vi "Ascan.vi"(8 "error in (no error)":cluster{"状态":bool, "代码":i32, "源":string} caption="错误输入（无错误）") -> (0 "error out":cluster{"状态":bool, "代码":i32, "源":string} caption="错误输出")   [LabVIEW 2015, in "Debug.lvlib"]
uses:
  Debug.lvlib
  Support/Debug Ascan UI Data.ctl
  Support/Ascan Configuration.ctl
  Sub VIs/DAQ/DAQ Configuration.ctl
  Sub VIs/Digital Signal Processing/Support/DSP Configuration.ctl
  <vilib>/Analysis/3filter.llb/Filter Passband Type.ctl
  <vilib>/Analysis/4window.llb/windowTd.ctl
  Sub VIs/Boimetry Processing/Controls/Biometry Configuration.ctl
  support/Message Queue/Enqueue Message (Single).vi
  <vilib>/Utility/error.llb/Error Cluster From Error Code.vi
  <vilib>/ErrorRing/Error Ring.xnode
  support/Message Queue/Message Queue.lvlib
  support/User Event - Stop/User Event - Stop.lvlib
  Sub VIs/DAQ/DAQ.lvlib
  <vilib>/Analysis/NI_AALBase.lvlib
  <vilib>/Analysis/NI_AALPro.lvlib
  Sub VIs/Digital Signal Processing/Digital Signal Processing.lvlib
  Sub VIs/Boimetry Processing/Boimetry Processing.lvlib
  Settings/Settings.lvlib
panel:
  in  "退出":bool
  in  "停止按钮":bool
  in  "计算距离":bool
  in  "保存按钮":bool
  in  "开始":bool
  in  "nd":dbl
  out "Thickness":dbl
  out "Position":dbl
  out "processing":dbl[](graph)
  out "original":i16[](graph)
  out "状态栏":string
  in  "Settings":bool
  in  "Liquid Len":bool
  in  "DSP Change":enum16{"1st", "2nd"}(ring)
  in  "WLED":bool
  in  "IRLED2":bool
  in  "IRLED1":bool
  in  "Motor":bool
  in  "SLD":bool
  # "Ascan Setting"
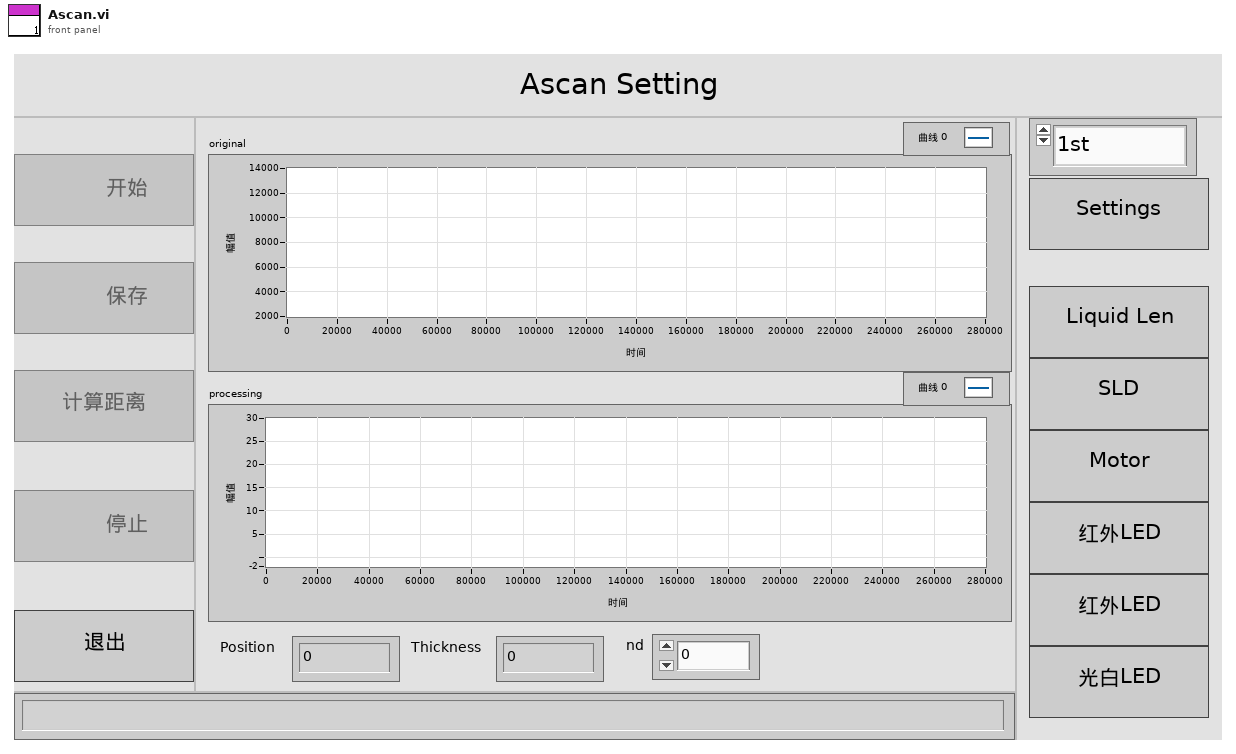
[diagram p1: front panel]
types:
  T1 = typedef "Debug.lvlib/Ascan Configuration.ctl" = cluster{"DAQ Configuration":T2, "DSP Parameter":T3, "Biometry Configuration":T6}
  T2 = typedef "DAQ.lvlib/DAQ Configuration.ctl" = cluster{"hDevice":i32, "DevNum":u8, "Configuration Parameter":i32[], "READ_MAX_LEN":i32, "DO":bool[]}
  T3 = typedef "Digital Signal Processing.lvlib/DSP Configuration.ctl" = cluster{"Sampling Frequency":dbl, "filter type":T4, "RF Filter Low Frequency":dbl, "RF Filter High Frequency":dbl, "RF Filter Taps":i32, "window":T5, "RF window parameter":dbl, "filter type 2":T4, "Demodulated Filter Low Frequency":dbl, "Demodulated Filter HighFrequency":dbl, "Demodulated Filter Order":i32, "SPAN":i32, "Logarithmic Base":dbl, "Noise path":string, "Work position parameter":i32[]}
  T4 = typedef "NI_AALBase.lvlib/Filter Passband Type.ctl" = enum32{"Lowpass", "Highpass", "Bandpass", "Bandstop"}
  T5 = typedef "NI_AALPro.lvlib/windowTd.ctl" = u32
  T6 = typedef "Boimetry Processing.lvlib/Biometry Configuration.ctl" = cluster{"Interference Width":i32, "Interference Threshold":dbl, "Cornea Len Division":i32, "Correction Data 1st Path":string, "1st_Start_Position":dbl, "Correction Data 2nd Path":string, "2nd_Start_Position":dbl, "Index Corneal":dbl, "Index Water":dbl, "Index Len":dbl, "Working Position":cluster{"FirstStart":i32, "FirstEnd":i32, "SecondStart":i32, "SecondEnd":i32}}
  T7 = typedef "Debug.lvlib/Debug Ascan UI Data.ctl" = cluster{"开始按钮引用句柄":refnum<vi>, "保持按钮引用句柄":refnum<vi>, "计算距离按钮l引用句柄":refnum<vi>, "停止按钮引用句柄":refnum<vi>, "状态栏引用句柄":refnum<vi>, "消息栏引用句柄":refnum<vi>, "退出按钮引用句柄":refnum<vi>, "SLD":refnum<vi>, "Motor":refnum<vi>}
  T8 = typedef "Message Queue.lvlib/All Message Queues Ascan.ctl" = cluster{"UI":refnum<queue>, "DAQ":refnum<queue>, "DSP":refnum<queue>, "CDL":refnum<queue>}
  T9 = typedef "Settings.lvlib/Settings.ctl" = cluster{"DAQ Configuration":T2, "DSP Configuration":T3, "Biometry Configuration":T6}
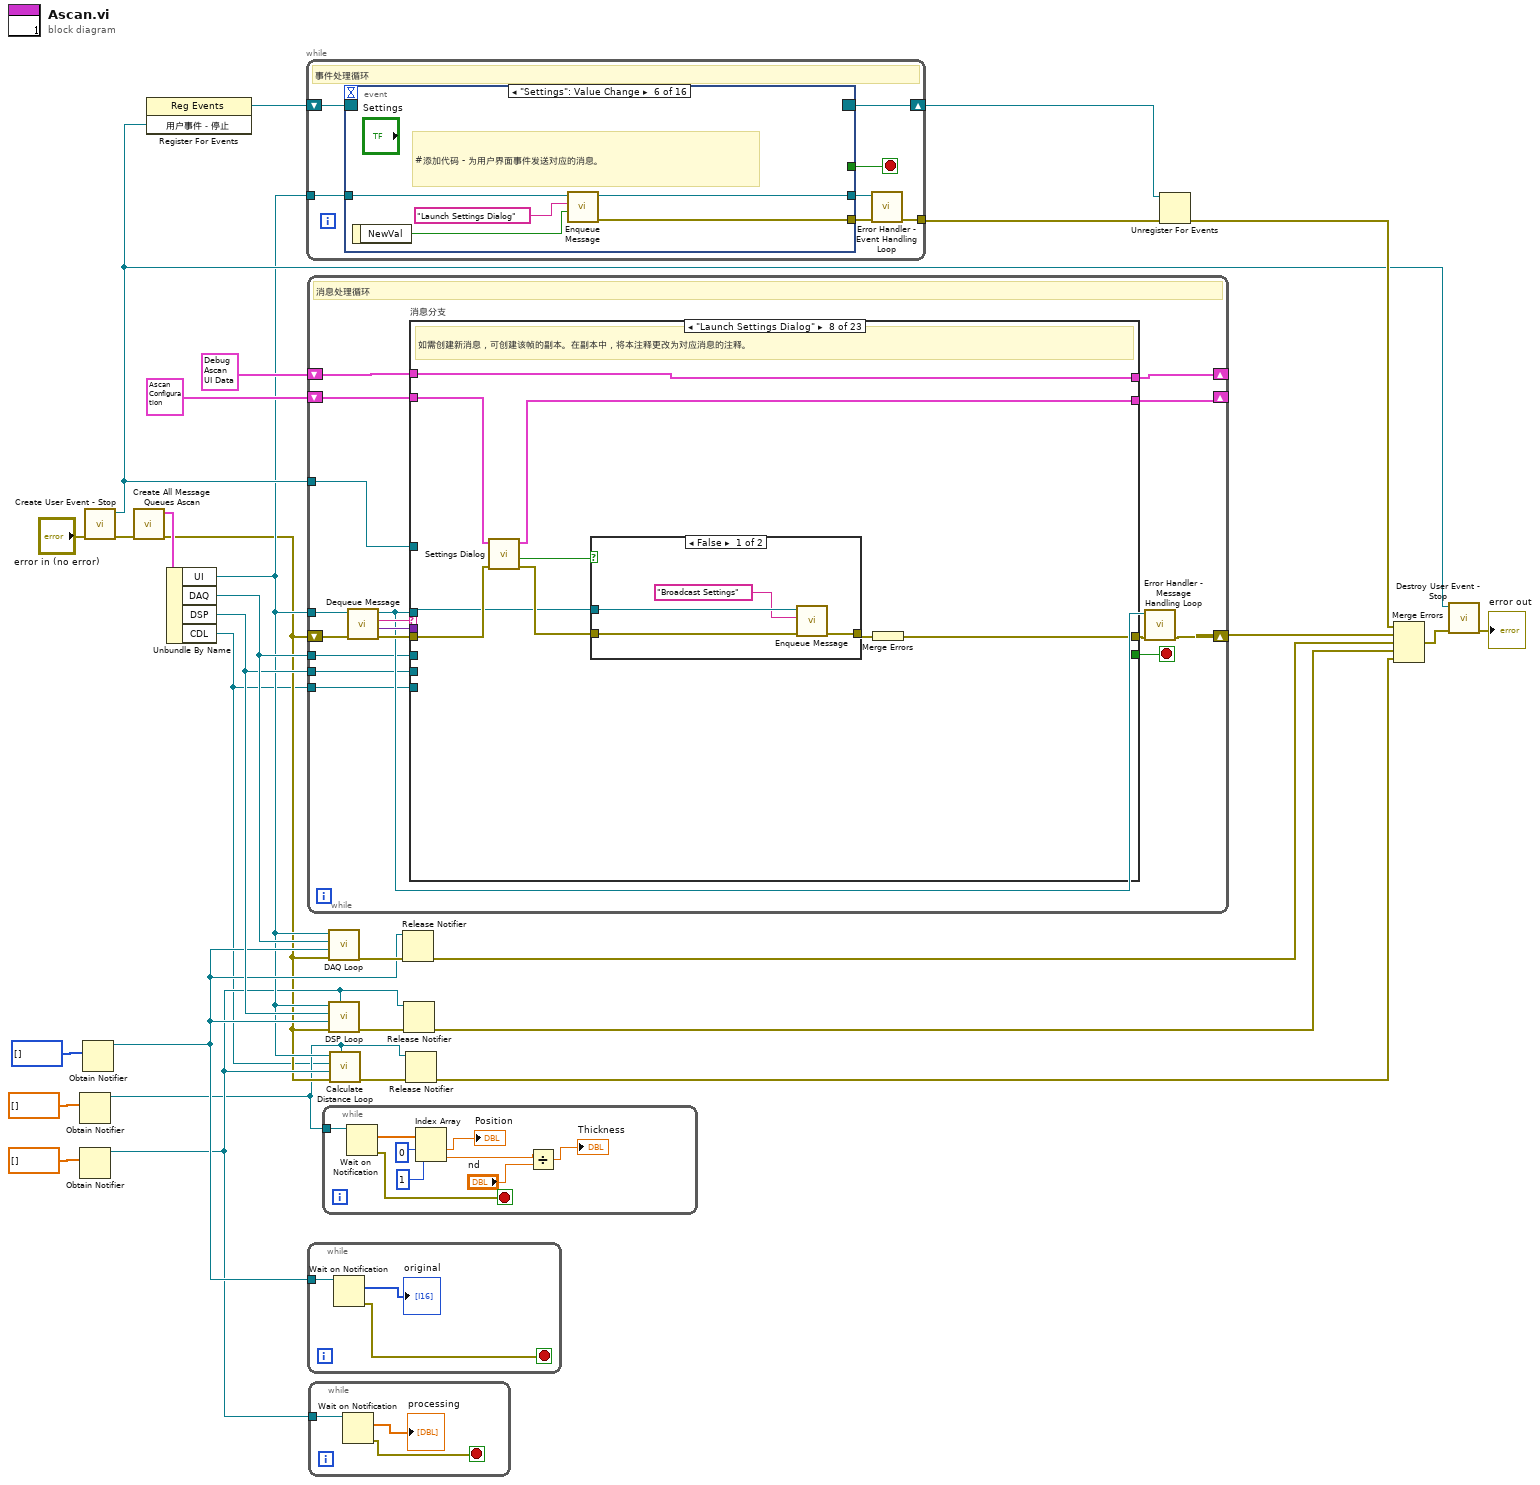
[diagram p0: block diagram]
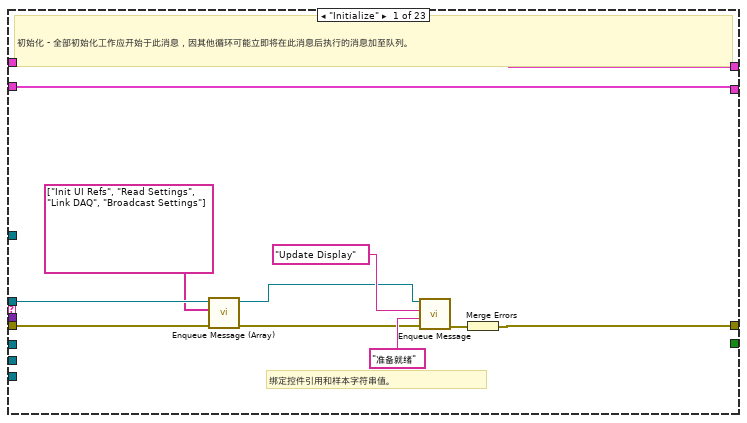
[diagram p2: hidden frame]
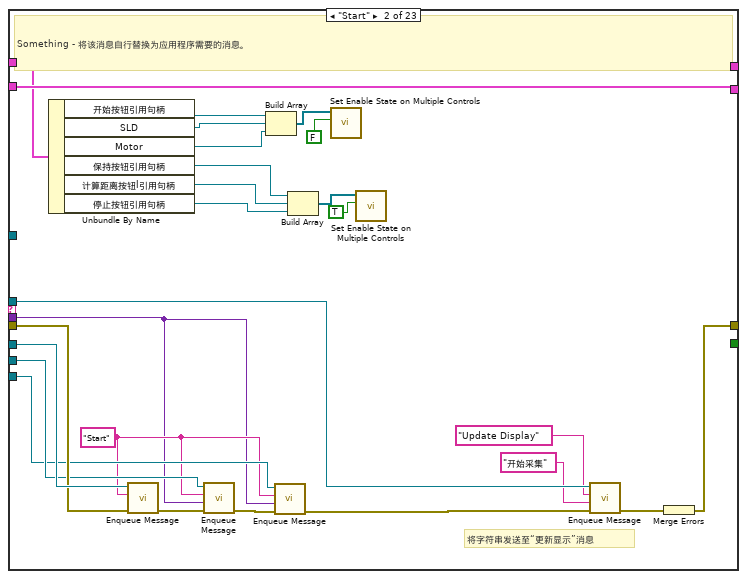
[diagram p3: hidden frame]
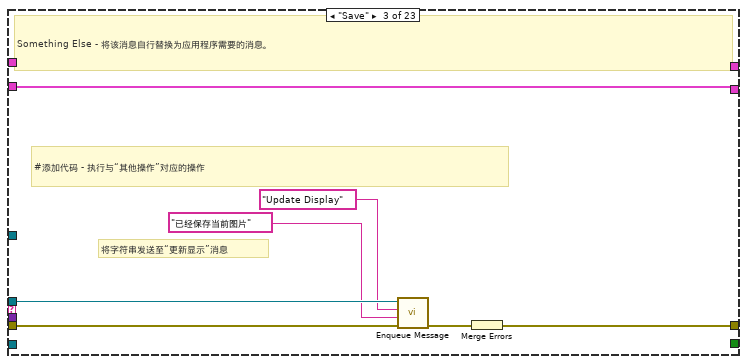
[diagram p4: hidden frame]
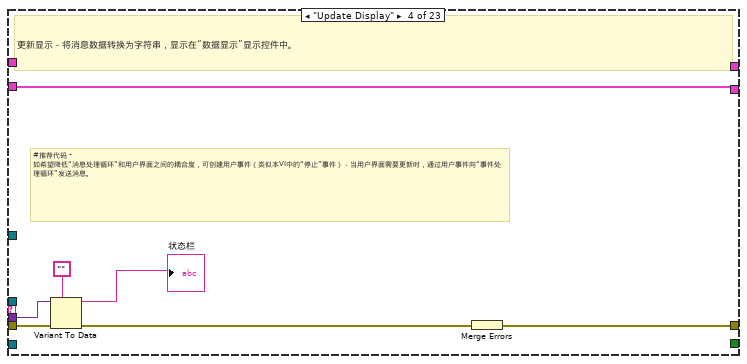
[diagram p5: hidden frame]
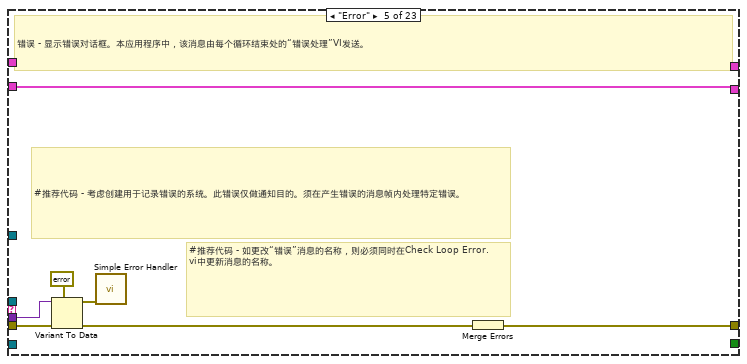
[diagram p6: hidden frame]
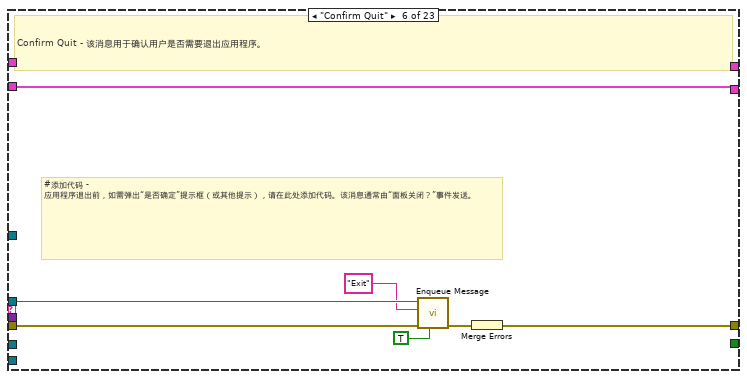
[diagram p7: hidden frame]
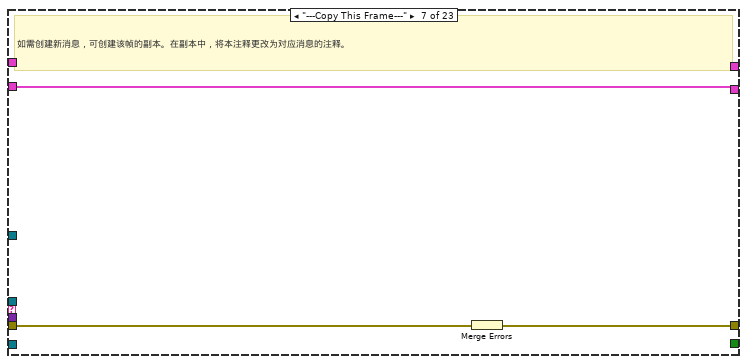
[diagram p8: hidden frame]
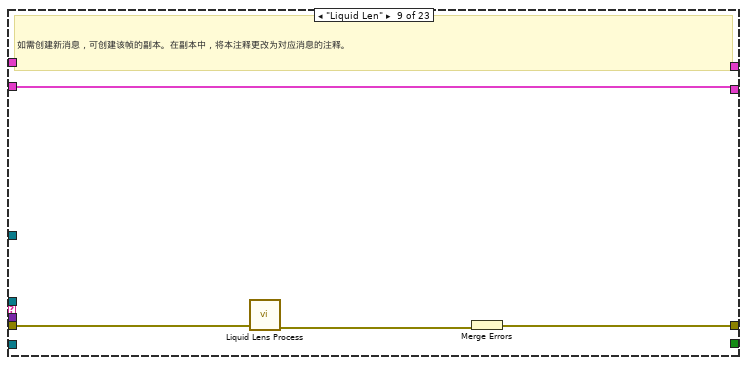
[diagram p10: hidden frame]
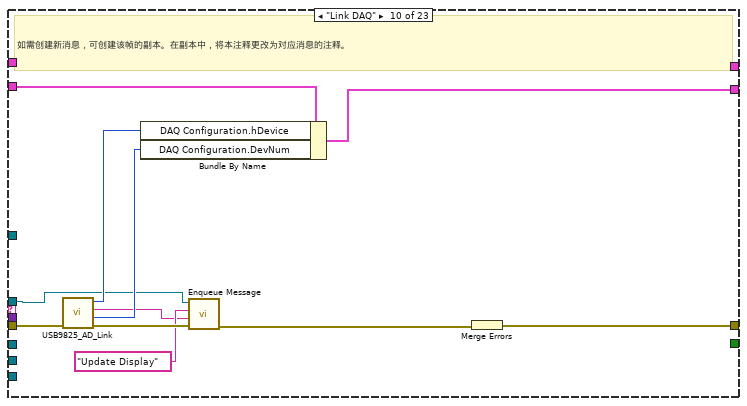
[diagram p11: hidden frame]
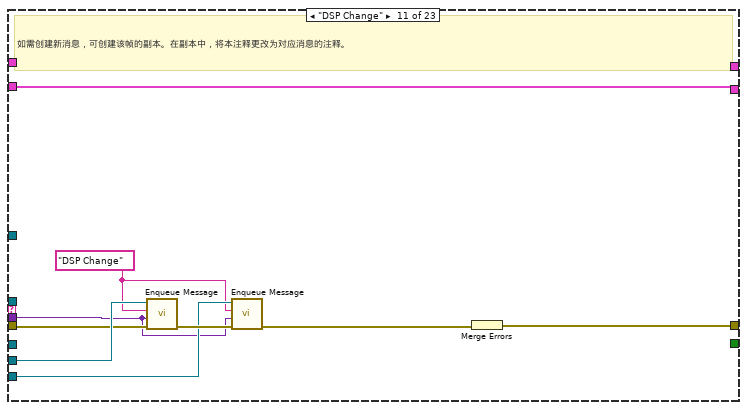
[diagram p12: hidden frame]
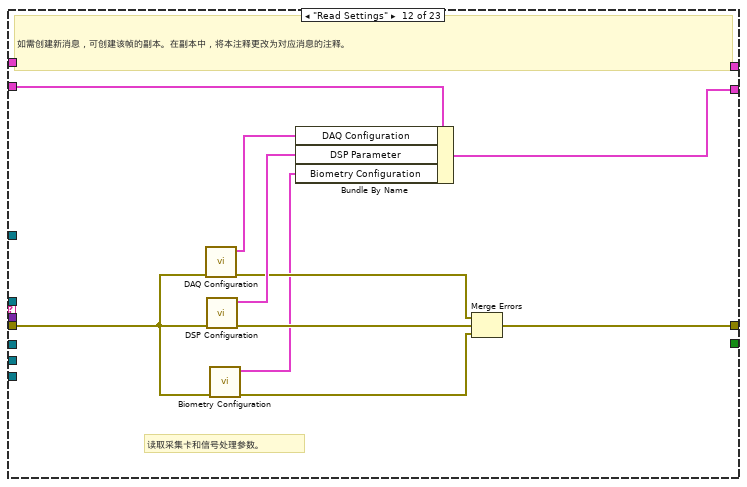
[diagram p13: hidden frame]
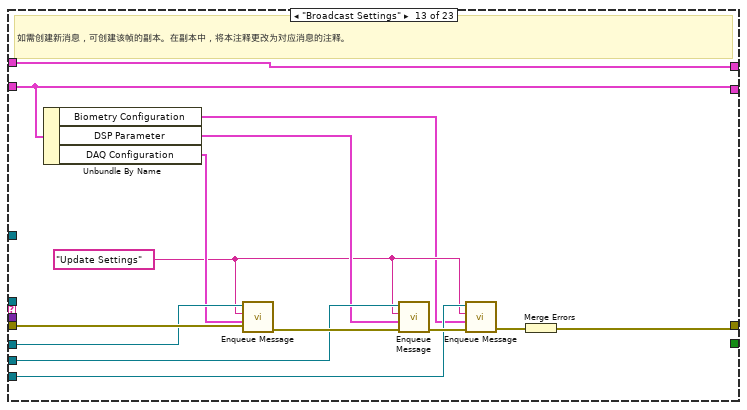
[diagram p14: hidden frame]
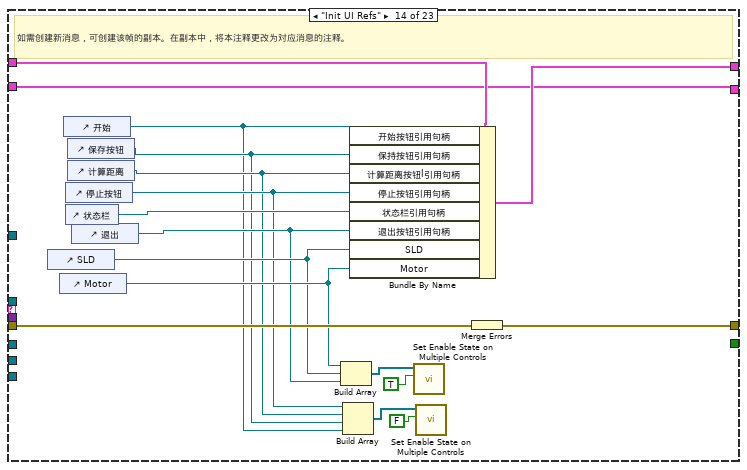
[diagram p15: hidden frame]
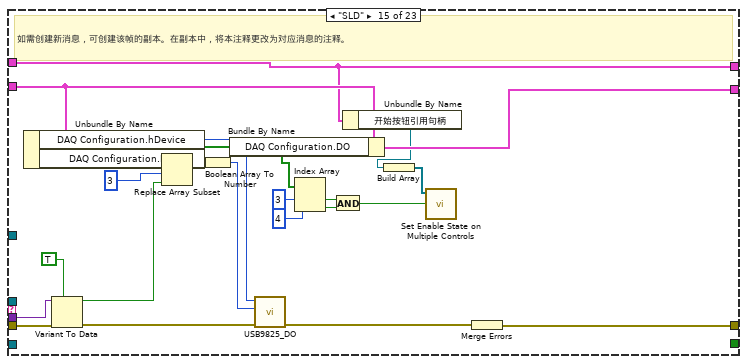
[diagram p16: hidden frame]
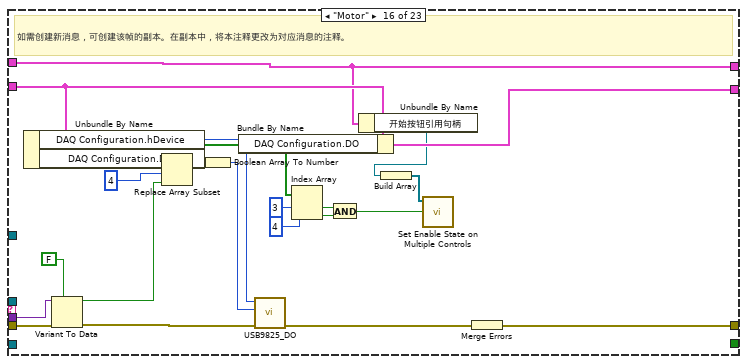
[diagram p17: hidden frame]
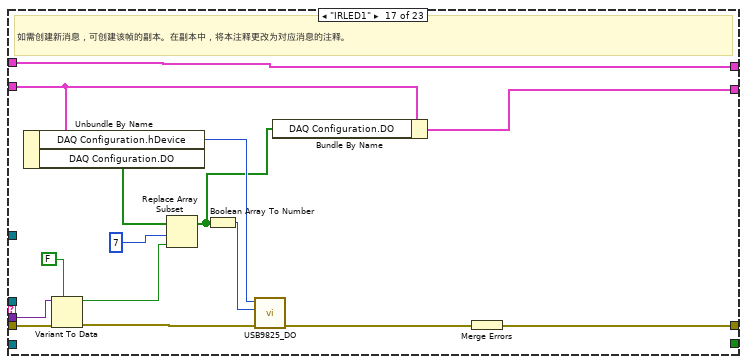
[diagram p18: hidden frame]
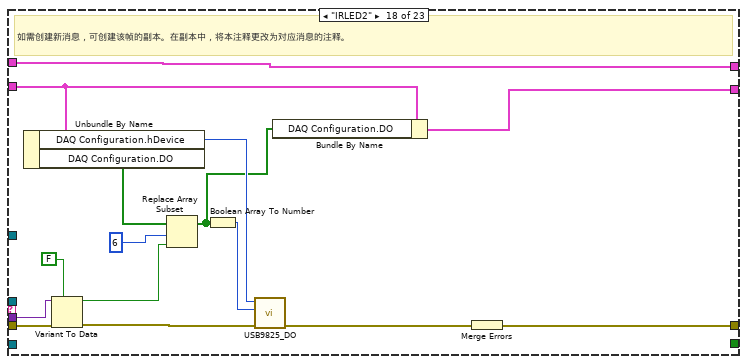
[diagram p19: hidden frame]
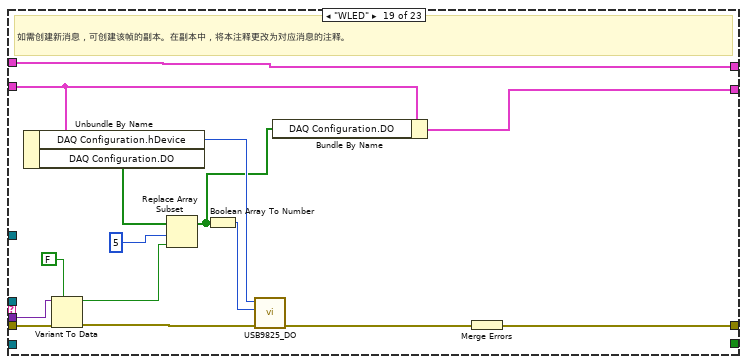
[diagram p20: hidden frame]
diagram:
  n1 = Obtain Notifier(notification data type=dbl[] []) -> (notifier out=w3:refnum<notifier>)  [unwired: 3 in, 2 out]
  n2 = Obtain Notifier(notification data type=dbl[] []) -> (notifier out=w7:refnum<notifier>)  [unwired: 3 in, 2 out]
  n3 = Obtain Notifier(notification data type=i16[] []) -> (notifier out=w12:refnum<notifier>)  [unwired: 3 in, 2 out]
  n4 = call "Create User Event - Stop.vi"("error in (no error)"="error in (no error)") -> ("error out"=w9:cluster{"状态":bool, "代码":i32, "源":string}, "用户事件－停止"=w25:refnum<user-event>)  [unwired: 9 in]
  n5 = call "Create All Message Queues Ascan.vi"("error in (no error)"=w9) -> ("error out"=w5:cluster{"状态":bool, "代码":i32, "源":string}, "消息队列"=w8:T8)  [unwired: 9 in]
  n6 = register-events(w25) -> (reference out=w30:refnum<event-registration>)  [unwired: 2 in, 1 out]
  n7 = Unbundle By Name(w8) -> ("UI"=w10:refnum<queue>, "DAQ"=w19:refnum<queue>, "DSP"=w14:refnum<queue>, "CDL"=w1:refnum<queue>)
  n8 = while {
    tunnel: w10 -> [w37]
    shift-right: [w35] -> w28
    shift-left: w30 -> [w36]
    tunnel: [w31] -> w29
    stop <- w33 stop-if-true
    # "事件处理循环"
    n9 = event shown="[5] \"Settings\": Value Change" {
      selector: w36 -> [_ _ _ _ _ _ _ _ _ _ _ _ _ _ _ _]
      dyn-events: [_ _ _ _ _ _ _ _ _ _ _ _ _ _ _ _] -> w35
      timeout: _ -> [_ _ _ _ _ _ _ _ _ _ _ _ _ _ _ _]
      tunnel: [_ _ _ _ _ _ _ _ _ _ _ _ _ _ _ TRUE ("Discard?")] -> w33
      tunnel: w37 -> [w43 w50 w56 w60 w65 w70 w75 w80 w85 w90 w95 w100 w102 w107 w112 w114]
      tunnel: [w40 _ w53 w57 w62 w67 w72 w77 w82 w87 w92 w99 _ w106 w111 _] -> w34
      tunnel: [w42 w49 w55 w59 w64 w69 w74 w79 w84 w89 w94 w98 w102 w105 w110 w114] -> w32
      event "开始": Value Change {
        n10 = event-data() -> ()  [unwired: 1 in, 1 out]
        n11 = local read "DSP Change"() -> (w39:enum16{"1st", "2nd"})
        n12 = case shown="\"2nd\"" w39 {
          tunnel: ["DSP 1st" ("Message") "DSP 2nd" ("Message")] -> w38
          frame "1st", Default {
          }
          frame "2nd" {
          }
        }
        n13 = call-poly "Enqueue Message.vi"("消息数据"=w38, "消息"="Start" ("Message"), "消息队列"=w43) -> ("error out"=w40:cluster{"状态":bool, "代码":i32, "源":string}, "消息队列副本"=w42:refnum<queue>)  [unwired: 7 in]
      }
      event "DSP Change": Value Change {
        n14 = event-data() -> ()  [unwired: 1 in, 1 out]
        n15 = case shown="\"2nd\"" "DSP Change" {
          tunnel: ["DSP 1st" ("Message") "DSP 2nd" ("Message")] -> w47
          frame "1st", Default {
          }
          frame "2nd" {
          }
        }
        n16 = call-poly "Enqueue Message.vi"("消息数据"=w47, "消息"="DSP Change", "消息队列"=w50) -> ("消息队列副本"=w49:refnum<queue>)  [unwired: 7 in, 1 out]
      }
      event "保存按钮": Value Change {
        # "#添加代码 - 为用户界面事件发送对应的消息。"
        n17 = event-data() -> ()  [unwired: 1 in, 1 out]
        n18 = call-poly "Enqueue Message.vi"("消息"="Save" ("Message"), "消息队列"=w56) -> ("error out"=w53:cluster{"状态":bool, "代码":i32, "源":string}, "消息队列副本"=w55:refnum<queue>)  [unwired: 8 in]
      }
      event "计算距离": Value Change {
        # "#添加代码 - 为用户界面事件发送对应的消息。"
        n19 = event-data() -> ()  [unwired: 1 in, 1 out]
        n20 = call-poly "Enqueue Message.vi"("消息"="Calculate" ("Message"), "消息队列"=w60) -> ("error out"=w57:cluster{"状态":bool, "代码":i32, "源":string}, "消息队列副本"=w59:refnum<queue>)  [unwired: 8 in]
      }
      event "SLD": Value Change {
        # "#添加代码 - 为用户界面事件发送对应的消息。"
        n21 = event-data() -> ("NewVal"=w61:bool)  [unwired: 1 in]
        n22 = call-poly "Enqueue Message.vi"("消息数据"=w61, "消息"="SLD" ("Message"), "消息队列"=w65) -> ("error out"=w62:cluster{"状态":bool, "代码":i32, "源":string}, "消息队列副本"=w64:refnum<queue>)  [unwired: 7 in]
      }
      event "Settings": Value Change {
        # "#添加代码 - 为用户界面事件发送对应的消息。"
        n23 = event-data() -> ("NewVal"=w66:bool)  [unwired: 1 in]
        n24 = call-poly "Enqueue Message.vi"("消息数据"=w66, "消息"="Launch Settings Dialog" ("Message"), "消息队列"=w70) -> ("error out"=w67:cluster{"状态":bool, "代码":i32, "源":string}, "消息队列副本"=w69:refnum<queue>)  [unwired: 7 in]
      }
      event "Motor": Value Change {
        # "#添加代码 - 为用户界面事件发送对应的消息。"
        n25 = event-data() -> ("NewVal"=w71:bool)  [unwired: 1 in]
        n26 = call-poly "Enqueue Message.vi"("消息数据"=w71, "消息"="Motor" ("Message"), "消息队列"=w75) -> ("error out"=w72:cluster{"状态":bool, "代码":i32, "源":string}, "消息队列副本"=w74:refnum<queue>)  [unwired: 7 in]
      }
      event "Liquid Len": Value Change {
        # "#添加代码 - 为用户界面事件发送对应的消息。"
        n27 = event-data() -> ("NewVal"=w76:bool)  [unwired: 1 in]
        n28 = call-poly "Enqueue Message.vi"("消息数据"=w76, "消息"="Liquid Len" ("Message"), "消息队列"=w80) -> ("error out"=w77:cluster{"状态":bool, "代码":i32, "源":string}, "消息队列副本"=w79:refnum<queue>)  [unwired: 7 in]
      }
      event "IRLED1": Value Change {
        # "#添加代码 - 为用户界面事件发送对应的消息。"
        n29 = event-data() -> ("NewVal"=w81:bool)  [unwired: 1 in]
        n30 = call-poly "Enqueue Message.vi"("消息数据"=w81, "消息"="IRLED1" ("Message"), "消息队列"=w85) -> ("error out"=w82:cluster{"状态":bool, "代码":i32, "源":string}, "消息队列副本"=w84:refnum<queue>)  [unwired: 7 in]
      }
      event "IRLED2": Value Change {
        # "#添加代码 - 为用户界面事件发送对应的消息。"
        n31 = event-data() -> ("NewVal"=w86:bool)  [unwired: 1 in]
        n32 = call-poly "Enqueue Message.vi"("消息数据"=w86, "消息"="IRLED2" ("Message"), "消息队列"=w90) -> ("error out"=w87:cluster{"状态":bool, "代码":i32, "源":string}, "消息队列副本"=w89:refnum<queue>)  [unwired: 7 in]
      }
      event "WLED": Value Change {
        # "#添加代码 - 为用户界面事件发送对应的消息。"
        n33 = event-data() -> ("NewVal"=w91:bool)  [unwired: 1 in]
        n34 = call-poly "Enqueue Message.vi"("消息数据"=w91, "消息"="WLED" ("Message"), "消息队列"=w95) -> ("error out"=w92:cluster{"状态":bool, "代码":i32, "源":string}, "消息队列副本"=w94:refnum<queue>)  [unwired: 7 in]
      }
      event Panel Close? {
        # "如用户关闭VI面板，则发送“确认退出”消息。丢弃事件，因此“确认退出”消息有运行时机。"
        n35 = event-data() -> ()  [unwired: 1 in, 1 out]
        n36 = call-poly "Enqueue Message.vi"("优先消息？ (F)"=TRUE ("Priority Message? (F)"), "消息"="Confirm Quit" ("Message"), "消息队列"=w100) -> ("error out"=w99:cluster{"状态":bool, "代码":i32, "源":string}, "消息队列副本"=w98:refnum<queue>)  [unwired: 7 in]
        n37 = event-data ("Event Filter Node")("Discard?"=TRUE) -> ()  [unwired: 1 in, 1 out]
      }
      event Application Instance Close {
        # "#推荐代码 - 当项目关闭时，项目的所有VI将被中止并从内存中释放。本事件帧内的所有代码都确保能够执行完成，因此可在此处添加必须执行的清理代码。"
        n38 = event-data() -> ()  [unwired: 1 in, 1 out]
      }
      event "停止按钮": Value Change {
        n39 = event-data() -> ()  [unwired: 1 in, 1 out]
        n40 = call-poly "Enqueue Message.vi"("优先消息？ (F)"=TRUE ("Priority Message? (F)"), "消息"="Stop" ("Message"), "消息队列"=w107) -> ("error out"=w106:cluster{"状态":bool, "代码":i32, "源":string}, "消息队列副本"=w105:refnum<queue>)  [unwired: 7 in]
      }
      event "退出": Value Change {
        n41 = event-data() -> ()  [unwired: 1 in, 1 out]
        n42 = call-poly "Enqueue Message.vi"("优先消息？ (F)"=TRUE ("Priority Message? (F)"), "消息"="Exit" ("Message"), "消息队列"=w112) -> ("error out"=w111:cluster{"状态":bool, "代码":i32, "源":string}, "消息队列副本"=w110:refnum<queue>)  [unwired: 7 in]
      }
      event User Event {
        (unwired) "“退出”按钮按下" ("VI Stopped")
        # "消息处理循环对“退出”消息进行处理，触发该事件，从而使事件处理循环停止运行。"
        n43 = event-data() -> ()  [unwired: 1 in, 1 out]
      }
    }
    n44 = call "Error Handler - Event Handling Loop.vi"("error in (no error)"=w34, "消息队列"=w32) -> ("错误输入副本"=w31:cluster{"状态":bool, "代码":i32, "源":string})  [unwired: 8 in, 1 out]
  }
  n45 = while {
    tunnel: w10 -> [w123]
    shift-right: [w130] -> _
    shift-left: T7 {"开始按钮引用句柄"=refnum, "保持按钮引用句柄"=refnum, "计算距离按钮l引用句柄"=refnum, "停止按钮引用句柄"=refnum, "状态栏引用句柄"=refnum, "消息栏引用句柄"=refnum, "退出按钮引用句柄"=refnum, "SLD"=refnum, "Motor"=refnum} ("UI数据") -> [w131]
    tunnel: w25 -> [w128]
    tunnel: w19 -> [w120]
    shift-right: [w118] -> _
    shift-left: T1 {"DAQ Configuration"={"hDevice"=0, "DevNum"=0, "Configuration Parameter"=[], "READ_MAX_LEN"=0, "DO"=[]}, "DSP Parameter"={"Sampling Frequency"=0.0, "filter type"=enum."Lowpass", "RF Filter Low Frequency"=0.0, "RF Filter High Frequency"=0.0, "RF Filter Taps"=0, "window"=0, "RF window parameter"=nan, "filter type 2"=enum."Lowpass", "Demodulated Filter Low Frequency"=0.0, "Demodulated Filter HighFrequency"=0.0, "Demodulated Filter Order"=0, "SPAN"=0, "Logarithmic Base"=0.0, "Noise path"="", "Work position parameter"=[]}, "Biometry Configuration"={"Interference Width"=0, "Interference Threshold"=0.0, "Cornea Len Division"=0, "Correction Data 1st Path"="", "1st_Start_Position"=0.0, "Correction Data 2nd Path"="", "2nd_Start_Position"=0.0, "Index Corneal"=0.0, "Index Water"=0.0, "Index Len"=0.0, "Working Position"={"FirstStart"=0, "FirstEnd"=0, "SecondStart"=0, "SecondEnd"=0}}} ("Ascan Configuration") -> [w119]
    tunnel: w14 -> [w117]
    shift-right: [w116] -> w18
    shift-left: w5 -> [w127]
    tunnel: w1 -> [w115]
    stop <- w129 stop-if-true
    # "消息处理循环"
    n46 = call "Dequeue Message.vi"("error in (no error)"=w127, "消息队列"=w123) -> ("error out"=w126:cluster{"状态":bool, "代码":i32, "源":string}, "消息数据"=w124:variant, "消息"=w125:string, "消息队列副本"=w122:refnum<queue>)  [unwired: 6 in]
    n47 = case "消息分支" shown="\"Launch Settings Dialog\"" w125 {
      selector: w125 -> [_ _ _ _ _ _ _ _ _ _ _ _ _ _ _ _ _ _ _ _ _ _ w420]
      tunnel: w122 -> [w137 w166 w172 _ _ w196 _ w206 _ w227 _ _ _ _ _ _ _ _ _ _ _ w418 _]
      tunnel: w126 -> [w134 w162 w174 w182 w192 w200 w204 w211 w220 w233 w241 w248 w268 w287 w308 w330 w345 w360 w375 w396 w401 w410 _]
      tunnel: [w139 w168 w175 w183 w186 w198 w202 w212 w222 w234 w244 w255 w269 w286 w309 w331 w346 w361 w376 w397 w399 w414 w421] -> w121
      tunnel: w131 -> [w138 w158 w176 w184 w191 w199 w203 w213 w223 w235 w245 w256 w270 w285 w291 w311 w332 w347 w362 w383 w400 w417 w422]
      tunnel: [w138 w158 w176 w184 w191 w199 w203 w213 w223 w235 w245 w256 w270 w284 w291 w311 w332 w347 w362 w383 w400 w417 w422] -> w130
      tunnel: [_ _ _ _ _ _ _ _ _ _ _ _ _ _ _ _ _ _ _ _ _ TRUE _] -> w129
      tunnel: w124 -> [_ w143 _ w181 w190 _ _ _ _ _ w236 _ _ _ w307 w329 w344 w359 w374 _ _ _ _]
      tunnel: w128 -> [_ _ _ _ _ _ _ _ _ _ _ _ _ _ _ _ _ _ _ _ _ w413 _]
      tunnel: w120 -> [_ w163 _ _ _ _ _ _ _ _ _ _ w267 _ _ _ _ _ _ w395 _ w411 _]
      tunnel: [w133 w161 w169 w177 w185 w193 w201 w209 w221 w224 w243 w251 w264 w271 w297 w319 w334 w349 w364 w394 w398 w409 w419] -> w118
      tunnel: w119 -> [w133 w161 w169 w177 w185 w193 w201 w210 w221 w232 w243 w252 w264 w271 w298 w320 w335 w350 w365 w394 w398 w409 w419]
      tunnel: w117 -> [_ w159 _ _ _ _ _ _ _ _ w242 _ w265 _ _ _ _ _ _ w392 _ w407 _]
      tunnel: w115 -> [_ w145 _ _ _ _ _ _ _ _ w238 _ w259 _ _ _ _ _ _ w378 _ w404 _]
      frame "Initialize" {
        # "绑定控件引用和样本字符串值。"
        # "初始化 - 全部初始化工作应开始于此消息，因其他循环可能立即将在此消息后执行的消息加至队列。"
        n48 = call "Enqueue Message (Array).vi"("error in (no error)"=w134, "消息数组"=string[] ["Init UI Refs", "Read Settings", "Link DAQ", "Broadcast Settings"], "消息队列"=w137) -> ("error out"=w132:cluster{"状态":bool, "代码":i32, "源":string}, "消息队列副本"=w136:refnum<queue>)  [unwired: 7 in]
        n49 = call-poly "Enqueue Message.vi"("error in (no error)"=w132, "消息数据"="准备就绪" ("Initial Message"), "消息"="Update Display" ("Message"), "消息队列"=w136) -> ("error out"=w140:cluster{"状态":bool, "代码":i32, "源":string})  [unwired: 6 in, 1 out]
        n50 = Merge Errors(w140) -> (w139:errorcluster)
      }
      frame "Start" {
        w144 = "Start" ("消息")
        # "将字符串发送至“更新显示”消息"
        # "Something - 将该消息自行替换为应用程序需要的消息。"
        n51 = Unbundle By Name(w158) -> ("开始按钮引用句柄"=w157:refnum<vi>, "SLD"=w149:refnum<vi>, "Motor"=w148:refnum<vi>, "保持按钮引用句柄"=w150:refnum<vi>, "计算距离按钮l引用句柄"=w151:refnum<vi>, "停止按钮引用句柄"=w152:refnum<vi>)
        n52 = call-poly "Enqueue Message.vi"("error in (no error)"=w162, "消息"=w144, "消息队列"=w163) -> ("error out"=w160:cluster{"状态":bool, "代码":i32, "源":string})  [unwired: 7 in, 1 out]
        n53 = call-poly "Enqueue Message.vi"("error in (no error)"=w160, "消息数据"=w143, "消息"=w144, "消息队列"=w159) -> ("error out"=w147:cluster{"状态":bool, "代码":i32, "源":string})  [unwired: 6 in, 1 out]
        n54 = Build Array(w157, w149, w148) -> (w156:refnum<vi>[])
        n55 = call-poly "Enqueue Message.vi"("error in (no error)"=w147, "消息数据"=w143, "消息"=w144, "消息队列"=w145) -> ("error out"=w146:cluster{"状态":bool, "代码":i32, "源":string})  [unwired: 6 in, 1 out]
        n56 = Build Array(w150, w151, w152) -> (w154:refnum<vi>[])
        n57 = call "Set Enable State on Multiple Controls.vi"("启用？"=FALSE, "控件"=w156) -> ()  [unwired: 10 in]
        n58 = call "Set Enable State on Multiple Controls.vi"("启用？"=TRUE, "控件"=w154) -> ()  [unwired: 10 in]
        n59 = call-poly "Enqueue Message.vi"("error in (no error)"=w146, "消息数据"="开始采集" ("\"Do Something\" button pressed"), "消息"="Update Display" ("Message"), "消息队列"=w166) -> ("error out"=w167:cluster{"状态":bool, "代码":i32, "源":string})  [unwired: 6 in, 1 out]
        n60 = Merge Errors(w167) -> (w168:errorcluster)
      }
      frame "Save" {
        # "将字符串发送至“更新显示”消息"
        # "#添加代码 - 执行与“其他操作”对应的操作"
        # "Something Else - 将该消息自行替换为应用程序需要的消息。"
        n61 = call-poly "Enqueue Message.vi"("error in (no error)"=w174, "消息数据"="已经保存当前图片" ("\"Do Something Else\" button pressed"), "消息"="Update Display" ("Message"), "消息队列"=w172) -> ("error out"=w173:cluster{"状态":bool, "代码":i32, "源":string})  [unwired: 6 in, 1 out]
        n62 = Merge Errors(w173) -> (w175:errorcluster)
      }
      frame "Update Display" {
        # "#推荐代码 - 如希望降低“消息处理循环”和用户界面之间的耦合度，可创建用户事件（类似本VI中的“停止”事件）－当用户界面需要更新时，通过用户事件向“事件处理循环”发送消息。"
        # "更新显示－将消息数据转换为字符串，显示在“数据显示”显示控件中。"
        n63 = Variant To Data(error in=w182, type="", Variant=w181) -> (data=→"状态栏":string, error out=w179:errorcluster)
        n64 = Merge Errors(w179) -> (w183:errorcluster)
      }
      frame "Error" {
        # "#推荐代码 - 如更改“错误”消息的名称，则必须同时在Check Loop Error.vi中更新消息的名称。"
        # "#推荐代码 - 考虑创建用于记录错误的系统。此错误仅做通知目的。须在产生错误的消息帧内处理特定错误。"
        # "错误 - 显示错误对话框。本应用程序中，该消息由每个循环结束处的“错误处理”VI发送。"
        n65 = Variant To Data(error in=w192, type=errorcluster {"status"=FALSE, "code"=0, "source"=""} ("error constant"), Variant=w190) -> (data=w188:errorcluster, error out=w187:errorcluster)
        n66 = call <vilib>:"Simple Error Handler.vi"("error in (no error)"=w188) -> ()  [unwired: 4 in, 5 out]
        n67 = Merge Errors(w187) -> (w186:errorcluster)
      }
      frame "Confirm Quit" {
        # "#添加代码 - 应用程序退出前，如需弹出“是否确定”提示框（或其他提示），请在此处添加代码。该消息通常由“面板关闭？”事件发送。"
        # "Confirm Quit - 该消息用于确认用户是否需要退出应用程序。"
        n68 = call-poly "Enqueue Message.vi"("优先消息？ (F)"=TRUE ("Priority Message? (F)"), "error in (no error)"=w200, "消息"="Exit" ("Message"), "消息队列"=w196) -> ("error out"=w197:cluster{"状态":bool, "代码":i32, "源":string})  [unwired: 6 in, 1 out]
        n69 = Merge Errors(w197) -> (w198:errorcluster)
      }
      frame "---Copy This Frame---" {
        # "如需创建新消息，可创建该帧的副本。在副本中，将本注释更改为对应消息的注释。"
        n70 = Merge Errors(w204) -> (w202:errorcluster)
      }
      frame "Launch Settings Dialog" {
        # "如需创建新消息，可创建该帧的副本。在副本中，将本注释更改为对应消息的注释。"
        n71 = call "Settings Dialog.vi"("error in (no error)"=w211, "Settings in"=w210) -> ("error out"=w208:errorcluster, "Cancelled?"=w207:bool, "Settings out"=w209:T9)  [unwired: 6 in, 1 out]
        n72 = case shown="False" w207 {
          tunnel: w206 -> [w217 _]
          tunnel: w208 -> [w216 w218]
          tunnel: [w215 w218] -> w205
          frame False {
            n73 = call-poly "Enqueue Message.vi"("error in (no error)"=w216, "消息"="Broadcast Settings" ("Message"), "消息队列"=w217) -> ("error out"=w215:cluster{"状态":bool, "代码":i32, "源":string})  [unwired: 7 in, 1 out]
          }
          frame True {
          }
        }
        n74 = Merge Errors(w205) -> (w212:errorcluster)
      }
      frame "Liquid Len" {
        # "如需创建新消息，可创建该帧的副本。在副本中，将本注释更改为对应消息的注释。"
        n75 = call "Liquid Lens Process.vi"("error in"=w220) -> ("error out"=w219:errorcluster)  [unwired: 10 in]
        n76 = Merge Errors(w219) -> (w222:errorcluster)
      }
      frame "Link DAQ" {
        # "如需创建新消息，可创建该帧的副本。在副本中，将本注释更改为对应消息的注释。"
        n77 = call "USB9825_AD_Link.vi"("Error In"=w233) -> ("Error Out"=w229:errorcluster, "DevNum"=w230:i32, "设备属性"=w225:string, "hDevice"=w231:i32)  [unwired: 7 in]
        n78 = Bundle By Name(cluster=w232, "DAQ Configuration.hDevice"=w231, "DAQ Configuration.DevNum"=w230) -> (w224:T1)
        n79 = call-poly "Enqueue Message.vi"("error in (no error)"=w229, "消息数据"=w225, "消息"="Update Display", "消息队列"=w227) -> ("error out"=w228:cluster{"状态":bool, "代码":i32, "源":string})  [unwired: 6 in, 1 out]
        n80 = Merge Errors(w228) -> (w234:errorcluster)
      }
      frame "DSP Change" {
        w237 = "DSP Change" ("消息")
        # "如需创建新消息，可创建该帧的副本。在副本中，将本注释更改为对应消息的注释。"
        n81 = call-poly "Enqueue Message.vi"("error in (no error)"=w241, "消息数据"=w236, "消息"=w237, "消息队列"=w242) -> ("error out"=w240:cluster{"状态":bool, "代码":i32, "源":string})  [unwired: 6 in, 1 out]
        n82 = call-poly "Enqueue Message.vi"("error in (no error)"=w240, "消息数据"=w236, "消息"=w237, "消息队列"=w238) -> ("error out"=w239:cluster{"状态":bool, "代码":i32, "源":string})  [unwired: 6 in, 1 out]
        n83 = Merge Errors(w239) -> (w244:errorcluster)
      }
      frame "Read Settings" {
        # "读取采集卡和信号处理参数。"
        # "如需创建新消息，可创建该帧的副本。在副本中，将本注释更改为对应消息的注释。"
        n84 = call "DAQ Configuration.vi"("error in (no error)"=w248) -> ("error out"=w249:errorcluster, "parameter output"=w254:T2)  [unwired: 9 in]
        n85 = call "DSP Configuration.vi"("error in (no error)"=w248) -> ("error out"=w250:errorcluster, "DSP Parameter Output"=w253:T3)  [unwired: 9 in]
        n86 = call "Biometry Configuration.vi"("error in (no error)"=w248) -> ("error out"=w247:errorcluster, "Biometry Configuration"=w246:T6)  [unwired: 9 in]
        n87 = Bundle By Name(cluster=w252, "DAQ Configuration"=w254, "DSP Parameter"=w253, "Biometry Configuration"=w246) -> (w251:T1)
        n88 = Merge Errors(w249, w250, w247) -> (w255:errorcluster)
      }
      frame "Broadcast Settings" {
        w258 = "Update Settings" ("消息")
        # "如需创建新消息，可创建该帧的副本。在副本中，将本注释更改为对应消息的注释。"
        n89 = Unbundle By Name(w264) -> ("Biometry Configuration"=w257:T6, "DSP Parameter"=w262:T3, "DAQ Configuration"=w263:T2)
        n90 = call-poly "Enqueue Message.vi"("error in (no error)"=w268, "消息数据"=w263, "消息"=w258, "消息队列"=w267) -> ("error out"=w266:cluster{"状态":bool, "代码":i32, "源":string})  [unwired: 6 in, 1 out]
        n91 = call-poly "Enqueue Message.vi"("error in (no error)"=w266, "消息数据"=w262, "消息"=w258, "消息队列"=w265) -> ("error out"=w260:cluster{"状态":bool, "代码":i32, "源":string})  [unwired: 6 in, 1 out]
        n92 = call-poly "Enqueue Message.vi"("error in (no error)"=w260, "消息数据"=w257, "消息"=w258, "消息队列"=w259) -> ("error out"=w261:cluster{"状态":bool, "代码":i32, "源":string})  [unwired: 6 in, 1 out]
        n93 = Merge Errors(w261) -> (w269:errorcluster)
      }
      frame "Init UI Refs" {
        # "如需创建新消息，可创建该帧的副本。在副本中，将本注释更改为对应消息的注释。"
        n94 = control-ref of="SLD"() -> (w281:refnum<vi>)
        n95 = control-ref of="Motor"() -> (w282:refnum<vi>)
        n96 = control-ref of="开始"() -> (w274:refnum<vi>)
        n97 = control-ref of="停止按钮"() -> (w277:refnum<vi>)
        n98 = control-ref of="状态栏"() -> (w283:refnum<vi>)
        n99 = control-ref of="保存按钮"() -> (w275:refnum<vi>)
        n100 = control-ref of="计算距离"() -> (w276:refnum<vi>)
        n101 = control-ref of="退出"() -> (w280:refnum<vi>)
        n102 = Build Array(w282, w281, w280) -> (w279:refnum<vi>[])
        n103 = Build Array(w277, w276, w275, w274) -> (w273:refnum<vi>[])
        n104 = Bundle By Name(cluster=w285, "开始按钮引用句柄"=w274, "保持按钮引用句柄"=w275, "计算距离按钮l引用句柄"=w276, "停止按钮引用句柄"=w277, "状态栏引用句柄"=w283, "退出按钮引用句柄"=w280, "SLD"=w281, "Motor"=w282) -> (w284:T7)
        n105 = call "Set Enable State on Multiple Controls.vi"("启用？"=TRUE, "控件"=w279) -> ()  [unwired: 10 in]
        n106 = call "Set Enable State on Multiple Controls.vi"("启用？"=FALSE, "控件"=w273) -> ()  [unwired: 10 in]
        n107 = Merge Errors(w287) -> (w286:errorcluster)
      }
      frame "SLD" {
        # "如需创建新消息，可创建该帧的副本。在副本中，将本注释更改为对应消息的注释。"
        n108 = Unbundle By Name(w298) -> ("DAQ Configuration.hDevice"=w301:i32, "DAQ Configuration.DO"=w305:bool[])
        n109 = Variant To Data(error in=w308, type=TRUE, Variant=w307) -> (data=w303:bool, error out=w300:errorcluster)
        n110 = Replace Array Subset(array=w305, new element=w303, index=3 ("索引")) -> (w292:bool[])
        n111 = Boolean Array To Number(Boolean array=w292) -> (number=w302:u32)
        n112 = Bundle By Name(cluster=w298, "DAQ Configuration.DO"=w292) -> (w297:T1)
        n113 = call "USB9825_DO.vi"("Error In"=w300, "pDO"=w302, "hDevice"=w301) -> ("Error Out"=w299:errorcluster)  [unwired: 8 in]
        n114 = Index Array(array=w292, index #1=3 ("索引"), index #2=4 ("索引")) -> (element #1=w293:bool, element #2=w294:bool)
        n115 = And(x=w293, y=w294) -> (x .and. y?=w290:bool)
        n116 = Unbundle By Name(w291) -> ("开始按钮引用句柄"=w289:refnum<vi>)
        n117 = Build Array(w289) -> (w288:refnum<vi>[])
        n118 = call "Set Enable State on Multiple Controls.vi"("启用？"=w290, "控件"=w288) -> ()  [unwired: 10 in]
        n119 = Merge Errors(w299) -> (w309:errorcluster)
      }
      frame "Motor" {
        # "如需创建新消息，可创建该帧的副本。在副本中，将本注释更改为对应消息的注释。"
        n120 = Unbundle By Name(w320) -> ("DAQ Configuration.hDevice"=w323:i32, "DAQ Configuration.DO"=w327:bool[])
        n121 = Variant To Data(error in=w330, type=FALSE, Variant=w329) -> (data=w325:bool, error out=w322:errorcluster)
        n122 = Replace Array Subset(array=w327, new element=w325, index=4 ("索引")) -> (w312:bool[])
        n123 = Boolean Array To Number(Boolean array=w312) -> (number=w324:u32)
        n124 = Bundle By Name(cluster=w320, "DAQ Configuration.DO"=w312) -> (w319:T1)
        n125 = call "USB9825_DO.vi"("Error In"=w322, "pDO"=w324, "hDevice"=w323) -> ("Error Out"=w321:errorcluster)  [unwired: 8 in]
        n126 = Index Array(array=w312, index #1=3 ("索引"), index #2=4 ("索引")) -> (element #1=w316:bool, element #2=w315:bool)
        n127 = And(x=w316, y=w315) -> (x .and. y?=w317:bool)
        n128 = Unbundle By Name(w311) -> ("开始按钮引用句柄"=w310:refnum<vi>)
        n129 = Build Array(w310) -> (w318:refnum<vi>[])
        n130 = call "Set Enable State on Multiple Controls.vi"("启用？"=w317, "控件"=w318) -> ()  [unwired: 10 in]
        n131 = Merge Errors(w321) -> (w331:errorcluster)
      }
      frame "IRLED1" {
        # "如需创建新消息，可创建该帧的副本。在副本中，将本注释更改为对应消息的注释。"
        n132 = Unbundle By Name(w335) -> ("DAQ Configuration.hDevice"=w338:i32, "DAQ Configuration.DO"=w342:bool[])
        n133 = Variant To Data(error in=w345, type=FALSE, Variant=w344) -> (data=w340:bool, error out=w337:errorcluster)
        n134 = Replace Array Subset(array=w342, new element=w340, index=7 ("索引")) -> (w333:bool[])
        n135 = Boolean Array To Number(Boolean array=w333) -> (number=w339:u32)
        n136 = call "USB9825_DO.vi"("Error In"=w337, "pDO"=w339, "hDevice"=w338) -> ("Error Out"=w336:errorcluster)  [unwired: 8 in]
        n137 = Bundle By Name(cluster=w335, "DAQ Configuration.DO"=w333) -> (w334:T1)
        n138 = Merge Errors(w336) -> (w346:errorcluster)
      }
      frame "IRLED2" {
        # "如需创建新消息，可创建该帧的副本。在副本中，将本注释更改为对应消息的注释。"
        n139 = Unbundle By Name(w350) -> ("DAQ Configuration.hDevice"=w353:i32, "DAQ Configuration.DO"=w357:bool[])
        n140 = Variant To Data(error in=w360, type=FALSE, Variant=w359) -> (data=w355:bool, error out=w352:errorcluster)
        n141 = Replace Array Subset(array=w357, new element=w355, index=6 ("索引")) -> (w348:bool[])
        n142 = Boolean Array To Number(Boolean array=w348) -> (number=w354:u32)
        n143 = call "USB9825_DO.vi"("Error In"=w352, "pDO"=w354, "hDevice"=w353) -> ("Error Out"=w351:errorcluster)  [unwired: 8 in]
        n144 = Bundle By Name(cluster=w350, "DAQ Configuration.DO"=w348) -> (w349:T1)
        n145 = Merge Errors(w351) -> (w361:errorcluster)
      }
      frame "WLED" {
        # "如需创建新消息，可创建该帧的副本。在副本中，将本注释更改为对应消息的注释。"
        n146 = Unbundle By Name(w365) -> ("DAQ Configuration.hDevice"=w368:i32, "DAQ Configuration.DO"=w372:bool[])
        n147 = Variant To Data(error in=w375, type=FALSE, Variant=w374) -> (data=w370:bool, error out=w367:errorcluster)
        n148 = Replace Array Subset(array=w372, new element=w370, index=5 ("索引")) -> (w363:bool[])
        n149 = Boolean Array To Number(Boolean array=w363) -> (number=w369:u32)
        n150 = call "USB9825_DO.vi"("Error In"=w367, "pDO"=w369, "hDevice"=w368) -> ("Error Out"=w366:errorcluster)  [unwired: 8 in]
        n151 = Bundle By Name(cluster=w365, "DAQ Configuration.DO"=w363) -> (w364:T1)
        n152 = Merge Errors(w366) -> (w376:errorcluster)
      }
      frame "Stop" {
        w377 = "Stop" ("消息")
        # "如需创建新消息，可创建该帧的副本。在副本中，将本注释更改为对应消息的注释。"
        n153 = Unbundle By Name(w383) -> ("开始按钮引用句柄"=w391:refnum<vi>, "SLD"=w382:refnum<vi>, "Motor"=w381:refnum<vi>, "保持按钮引用句柄"=w386:refnum<vi>, "计算距离按钮l引用句柄"=w385:refnum<vi>, "停止按钮引用句柄"=w384:refnum<vi>)
        n154 = call-poly "Enqueue Message.vi"("error in (no error)"=w396, "消息"=w377, "消息队列"=w395) -> ("error out"=w393:cluster{"状态":bool, "代码":i32, "源":string})  [unwired: 7 in, 1 out]
        n155 = call-poly "Enqueue Message.vi"("error in (no error)"=w393, "消息"=w377, "消息队列"=w392) -> ("error out"=w380:cluster{"状态":bool, "代码":i32, "源":string})  [unwired: 7 in, 1 out]
        n156 = Build Array(w391, w382, w381) -> (w390:refnum<vi>[])
        n157 = call-poly "Enqueue Message.vi"("error in (no error)"=w380, "消息"=w377, "消息队列"=w378) -> ("error out"=w379:cluster{"状态":bool, "代码":i32, "源":string})  [unwired: 7 in, 1 out]
        n158 = Build Array(w386, w385, w384) -> (w388:refnum<vi>[])
        n159 = call "Set Enable State on Multiple Controls.vi"("启用？"=TRUE, "控件"=w390) -> ()  [unwired: 10 in]
        n160 = call "Set Enable State on Multiple Controls.vi"("启用？"=FALSE, "控件"=w388) -> ()  [unwired: 10 in]
        n161 = Merge Errors(w379) -> (w397:errorcluster)
      }
      frame "Calculate" {
        # "如需创建新消息，可创建该帧的副本。在副本中，将本注释更改为对应消息的注释。"
        n162 = Merge Errors(w401) -> (w399:errorcluster)
      }
      frame "Exit" {
        w402 = TRUE ("优先消息？ (F)")
        w403 = "Exit" ("消息")
        # "停止VI"
        # "释放消息队列引用"
        # "#添加代码 - 此处按需要添加清理代码。注意，如果'退出' 作为错误结果被调用，则将显示错误对话框。为“退出”条件添加自定义错误处理。"
        # "退出 - 退出应用程序。"
        n163 = call-poly "Enqueue Message.vi"("优先消息？ (F)"=w402, "error in (no error)"=w410, "消息"=w403, "消息队列"=w411) -> ("error out"=w408:cluster{"状态":bool, "代码":i32, "源":string})  [unwired: 6 in, 1 out]
        n164 = Release Queue(queue=w418, error in (no error)=w410) -> (error out=w415:errorcluster)  [unwired: 1 in, 2 out]
        n165 = call-poly "Enqueue Message.vi"("优先消息？ (F)"=w402, "error in (no error)"=w408, "消息"=w403, "消息队列"=w407) -> ("error out"=w406:cluster{"状态":bool, "代码":i32, "源":string})  [unwired: 6 in, 1 out]
        n166 = call-poly "Enqueue Message.vi"("优先消息？ (F)"=w402, "error in (no error)"=w406, "消息"=w403, "消息队列"=w404) -> ("error out"=w405:cluster{"状态":bool, "代码":i32, "源":string})  [unwired: 6 in, 1 out]
        n167 = call "Fire User Event - Stop.vi"("用户事件－停止"=w413) -> ("error out"=w412:cluster{"状态":bool, "代码":i32, "源":string})  [unwired: 10 in]
        n168 = Merge Errors(w412, w415, w405) -> (w414:errorcluster)
      }
      frame Default {
        # "如得到的消息未经任何分支定义，则运行“默认”分支。输出程序错误。"
        n169 = xnode ("Error Ring")("parameter 0"=w420) -> ("error out"=w421:errorcluster)
      }
    }
    n170 = call "Error Handler - Message Handling Loop.vi"("error in (no error)"=w121, "消息队列"=w122) -> ("错误输入副本"=w116:cluster{"状态":bool, "代码":i32, "源":string})  [unwired: 8 in, 1 out]
  }
  n171 = while {
    tunnel: w12 -> [w432]
    stop <- w430 stop-if-true
    n172 = Wait on Notification(notifier=w432) -> (notification=→"original":i16[], error out=w430:errorcluster)  [unwired: 3 in, 2 out]
  }
  n173 = while {
    tunnel: w7 -> [w433]
    stop <- w435 stop-if-true
    n174 = Wait on Notification(notifier=w433) -> (notification=→"processing":dbl[], error out=w435:errorcluster)  [unwired: 3 in, 2 out]
  }
  n175 = while {
    tunnel: w3 -> [w443]
    stop <- w444 stop-if-true
    n176 = Wait on Notification(notifier=w443) -> (notification=w442:dbl[], error out=w444:errorcluster)  [unwired: 3 in, 2 out]
    n177 = Index Array(array=w442, index #1=0 ("索引"), index #2=1 ("索引")) -> (element #1=→"Position":dbl, element #2=w437:dbl)
    n178 = Divide(x=w437, y="nd") -> (x/y=→"Thickness":dbl)
  }
  n179 = call "DAQ Loop.vi"("error in (no error)"=w5, "数据通知器"=w12, "DAQ"=w19, "Director"=w10) -> ("error out"=w17:errorcluster)  [unwired: 7 in]
  n180 = call "DSP Loop.vi"("数据通知器处理"=w7, "error in (no error)"=w5, "数据通知器原始"=w12, "DSP"=w14, "Director"=w10) -> ("error out"=w13:errorcluster)  [unwired: 6 in]
  n181 = call "Calculate Distance Loop.vi"("Position And Thickness"=w3, "error in (no error)"=w5, "DSP Signal"=w7, "CDL"=w1, "Director"=w10) -> ("error out"=w4:errorcluster)  [unwired: 6 in]
  n182 = Release Notifier(notifier=w12, error in (no error)=w17) -> (error out=w16:errorcluster)  [unwired: 1 in, 2 out]
  n183 = Release Notifier(notifier=w7, error in (no error)=w13) -> (error out=w11:errorcluster)  [unwired: 1 in, 2 out]
  n184 = Release Notifier(notifier=w3, error in (no error)=w4) -> (error out=w2:errorcluster)  [unwired: 1 in, 2 out]
  n185 = Unregister For Events(event registration refnum=w28, error in=w29) -> (error out=w27:errorcluster)
  n186 = Merge Errors(w27, w18, w16, w11, w2) -> (w26:errorcluster)
  n187 = call "Destroy User Event - Stop.vi"("error in (no error)"=w26, "用户事件－停止"=w25) -> ("error out"=→"error out":cluster{"状态":bool, "代码":i32, "源":string})  [unwired: 9 in]
